vi "preprocessamento.vi"() -> (2 "Timestemp":dbl[](array[numeric]), 3 "Tensão B":dbl[](array[numeric]), 4 "Corrente B":dbl[](array[numeric]), 5 "Potência ativa B":dbl[](array[numeric]), 6 "Tensao C":dbl[](array[numeric]), 7 "Corrente C":dbl[](array[numeric]), 8 "Potência ativa C":dbl[](array[numeric]), 9 "Tensão  A":dbl[](array[numeric]), 10 "Corrente A":dbl[](array[numeric]), 11 "Potência ativa A":dbl[](array[numeric]))   [LabVIEW 2026]
uses:
  <vilib>/numeric/Random Number (Range) DBL.vi
panel:
  out "Waveform Chart":dbl(graph)
  out "Waveform Graph 3":dbl[](graph)
  out "Waveform Graph 2":dbl[](graph)
  out "Fator Potência":dbl
  out "Waveform Graph":dbl[](graph)
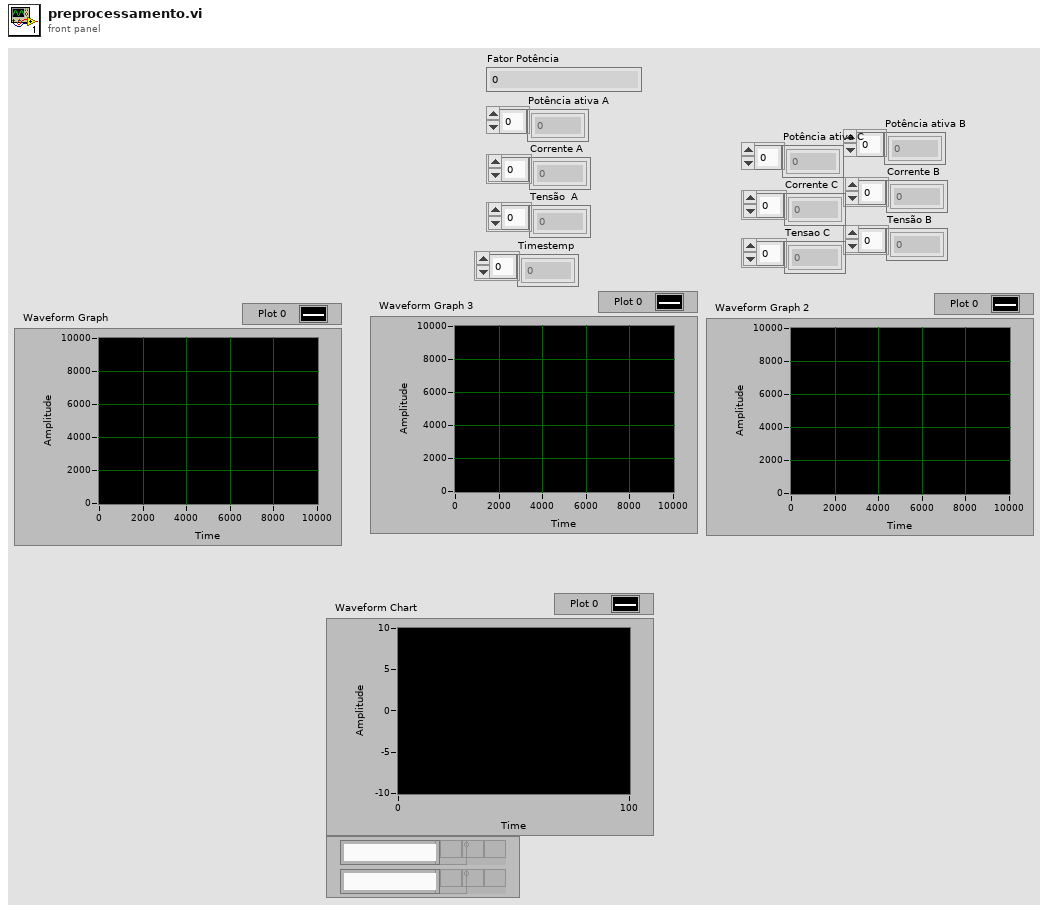
[diagram p1: front panel]
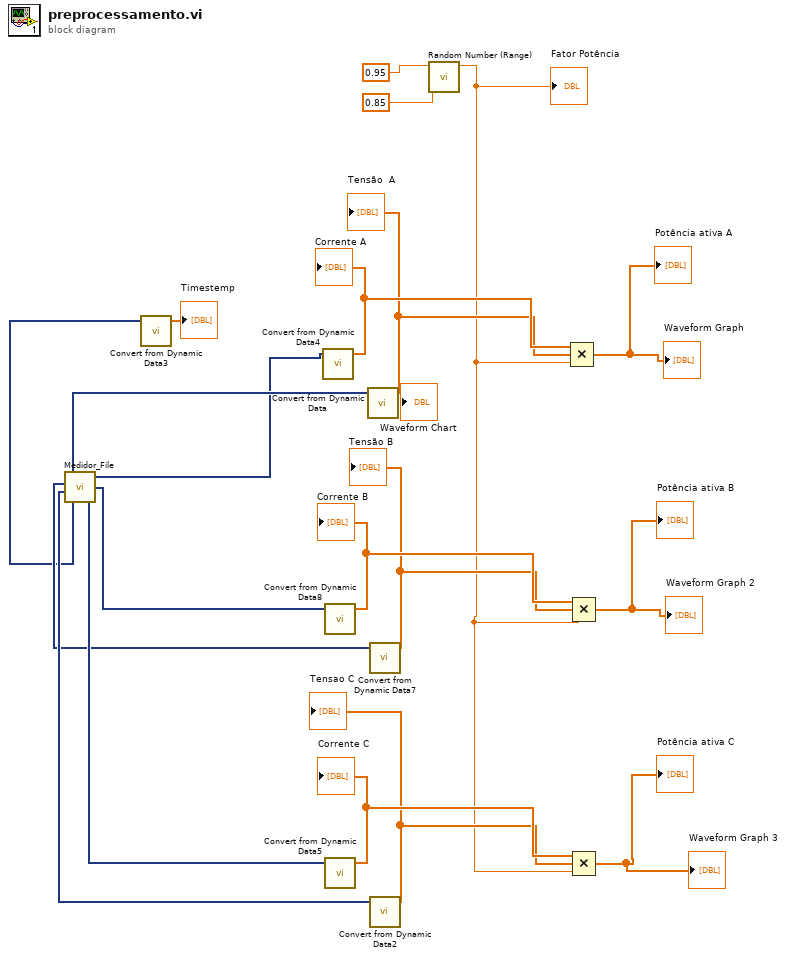
[diagram p0: block diagram]
diagram:
  n1 = call "Medidor_File.vi"() -> ("Corrente Fase C"=w6:dynamicdata, "Corrente Fase B"=w7:dynamicdata, "Corrente Fase A"=w8:dynamicdata, "TimeStamp"=w2:dynamicdata, "Tensão Fase C"=w5:dynamicdata, "Tensão Fase B"=w4:dynamicdata, "Tensão Fase A"=w9:dynamicdata)
  n2 = call "Convert from Dynamic Data3"("Dynamic Data Type"=w2) -> ("Array"=→"Timestemp":dbl[])  [unwired: 3 in]
  n3 = call "Convert from Dynamic Data4"("Dynamic Data Type"=w8) -> ("Array"=w17:dbl[])  [unwired: 3 in]
  "Corrente A" <- w17
  n4 = call "Convert from Dynamic Data8"("Dynamic Data Type"=w7) -> ("Array"=w14:dbl[])  [unwired: 3 in]
  "Corrente B" <- w14
  n5 = call "Convert from Dynamic Data5"("Dynamic Data Type"=w6) -> ("Array"=w12:dbl[])  [unwired: 3 in]
  "Corrente C" <- w12
  n6 = call "Convert from Dynamic Data"("Dynamic Data Type"=w9) -> ("Array"=w16:dbl[])  [unwired: 3 in]
  "Tensão  A" <- w16
  n7 = call "Convert from Dynamic Data7"("Dynamic Data Type"=w4) -> ("Array"=w13:dbl[])  [unwired: 3 in]
  "Tensão B" <- w13
  n8 = call "Convert from Dynamic Data2"("Dynamic Data Type"=w5) -> ("Array"=w11:dbl[])  [unwired: 3 in]
  "Tensao C" <- w11
  n9 = call-poly <vilib>:"Random Number (Range).vi"("lower bound (0)"=0.85, "upper bound (100)"=0.95) -> ("number"=w10:dbl)  [unwired: 9 in]
  "Fator Potência" <- w10
  n10 = Compound Arithmetic op=MULTIPLY(w17, w16, w10) -> (→"Waveform Graph" →"Potência ativa A":dbl[])
  n11 = Compound Arithmetic op=MULTIPLY(w14, w13, w10) -> (→"Waveform Graph 2" →"Potência ativa B":dbl[])
  n12 = Compound Arithmetic op=MULTIPLY(w12, w11, w10) -> (→"Potência ativa C" →"Waveform Graph 3":dbl[])
